vi "getConfigFilePath.vi"(8 "error in (no error)":errorcluster, 11 "reference in":refnum<class "File Controller.lvclass">) -> (0 "error out":errorcluster, 3 "reference out":refnum<class "File Controller.lvclass">)   [LabVIEW 2015, in "File Controller.lvclass"]
uses:
  File Controller.lvclass
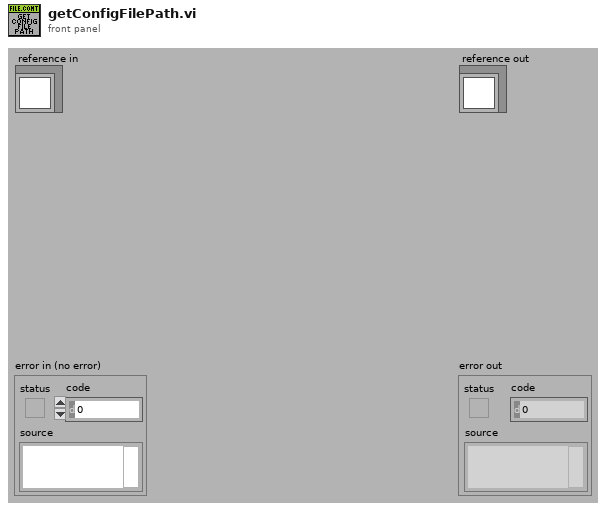
[diagram p1: front panel]
types:
  T1 = typedef "File Controller.lvclass/ObjectAttributesRef.ctl" = refnum<data-value>
  T2 = typedef "File Controller.lvclass/ObjectAttributes.ctl" = cluster{"MyAttribute":dbl, "excelFile_refs":refnum<class "excelFile.lvclass">[], "filePaths":path[], "outlookTemplatePaths":path[], "attachmentTemplatePaths":path[], "configFilePath":path, "not_setting":bool[], "python_ref":refnum<class "python.lvclass">}
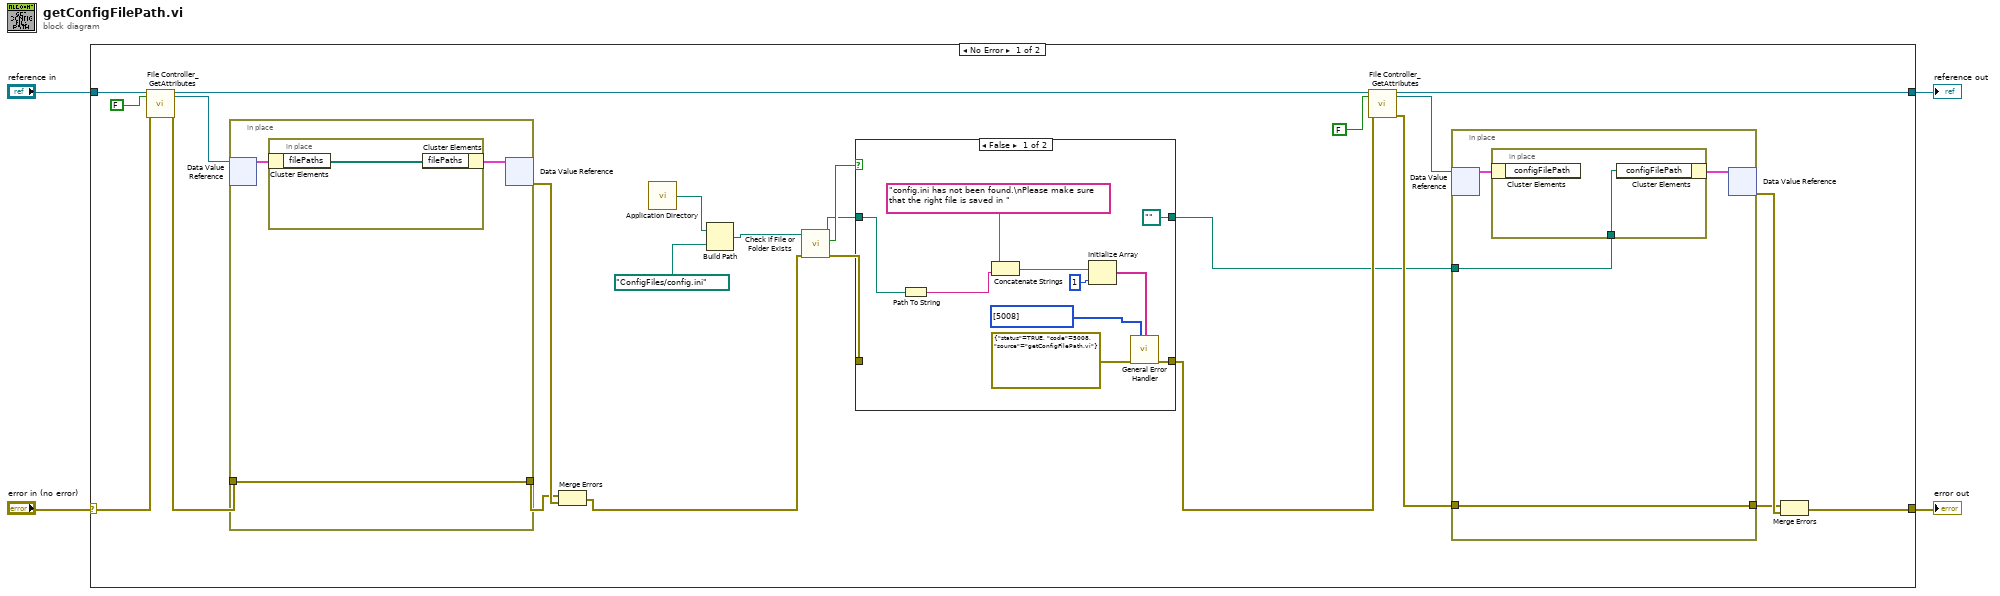
[diagram p0: block diagram]
diagram:
  n1 = case shown="No Error" "error in (no error)" {
    selector: "error in (no error)" -> [w24 w51]
    tunnel: [w8 w51] -> w3
    tunnel: [w6 w50] -> w1
    tunnel: "reference in" -> [w26 w50]
    frame No Error {
      n2 = call "File Controller_GetAttributes.vi"("reference in"=w26, "return data? (T)"=FALSE, "error in (no error)"=w24) -> ("reference out"=w7:refnum<class "File Controller.lvclass">, "attributes ref"=w22:T1, "error out"=w23:errorcluster)  [unwired: 13 in, 1 out]
      n3 = in-place {
        in-place-border: w23 -> [w46]
        in-place-border: [w46] -> w27
        n4 = in-place-dvr #1(w22) -> (w47:T2)  [unwired: 1 out]
        n5 = in-place {
          n6 = in-place-cluster #2(w47) -> ("filePaths"=w49:path[])
          n7 = in-place-cluster #2("filePaths"=w49) -> (w48:T2)
        }
        n8 = in-place-dvr #1(w48) -> (w28:errorcluster)  [unwired: 1 out]
      }
      n9 = Merge Errors(w27, w28) -> (w15:errorcluster)
      n10 = call <vilib>:"Application Directory.vi"() -> ("Application Directory"=w18:path)
      n11 = Build Path(base path=w18, name or relative path=path "ConfigFiles/config.ini" ("path")) -> (appended path=w17:path)
      n12 = call <vilib>:"Check if File or Folder Exists.vi"("error in (no error)"=w15, "path"=w17) -> ("error out"=w21:errorcluster, "file or folder exists?"=w20:bool, "dup path"=w16:path)  [unwired: 7 in]
      n13 = case shown="False" w20 {
        tunnel: w21 -> [_ w45]
        tunnel: [w43 w45] -> w9
        tunnel: w16 -> [w40 w44]
        tunnel: [path "" ("dup path") w44] -> w5
        frame False {
          n14 = Path To String(path=w40) -> (string=w36:string)
          n15 = Concatenate Strings("config.ini has not been found.\nPlease make sure that the right file is saved in ", w36) -> (w35:string)
          n16 = Initialize Array(w35, 1 ("dimension size")) -> (w39:string[])
          n17 = call <vilib>:"General Error Handler.vi"("[user-defined codes]"=i32[] [5008], "[user-defined descriptions]"=w39, "error in (no error)"=errorcluster {"status"=TRUE, "code"=5008, "source"="getConfigFilePath.vi"}) -> ("error out"=w43:errorcluster)  [unwired: 8 in, 4 out]
        }
        frame True {
        }
      }
      n18 = call "File Controller_GetAttributes.vi"("reference in"=w7, "return data? (T)"=FALSE, "error in (no error)"=w9) -> ("reference out"=w6:refnum<class "File Controller.lvclass">, "attributes ref"=w10:T1, "error out"=w11:errorcluster)  [unwired: 13 in, 1 out]
      n19 = in-place {
        in-place-border: w11 -> [w30]
        in-place-border: [w30] -> w13
        in-place-border: w5 -> [w29]
        n20 = in-place-dvr #3(w10) -> (w31:T2)  [unwired: 1 out]
        n21 = in-place {
          in-place-border: w29 -> [w33]
          n22 = in-place-cluster #4(w31) -> ()  [unwired: 1 out]
          n23 = in-place-cluster #4("configFilePath"=w33) -> (w32:T2)
        }
        n24 = in-place-dvr #3(w32) -> (w14:errorcluster)  [unwired: 1 out]
      }
      n25 = Merge Errors(w13, w14) -> (w8:errorcluster)
    }
    frame Error {
    }
  }
  "error out" <- w3
  "reference out" <- w1
